vi "bumper.vi"() -> ()   [LabVIEW 2013]
uses:
  E:/All_Physics/PRISM/Abadines/bumper.ctl
  <vilib>/NXT/Block Support/NXT_InputPort.ctl
  <vilib>/NXT/Subs/MotorOutput.ctl
panel:
  out "F.  Right":bool
  out "F. Left":bool
  out "Output Ports (A & B) 8":T1=4 items=["Port A"=0, "Port B"=1, "Port C"=2, "Ports A & B"=4, "Ports A & C"=5, "Ports B & C"=6, "All Ports"=3]
  out "Output Port (All Ports) 2":T1=3 items=["Port A"=0, "Port B"=1, "Port C"=2, "Ports A & B"=4, "Ports A & C"=5, "Ports B & C"=6, "All Ports"=3]
  out "Output Ports (A & B) 7":T1=4 items=["Port A"=0, "Port B"=1, "Port C"=2, "Ports A & B"=4, "Ports A & C"=5, "Ports B & C"=6, "All Ports"=3]
  out "Output Ports (A & B) 6":T1=4 items=["Port A"=0, "Port B"=1, "Port C"=2, "Ports A & B"=4, "Ports A & C"=5, "Ports B & C"=6, "All Ports"=3]
  out "Output Ports (A & B) 5":T1=4 items=["Port A"=0, "Port B"=1, "Port C"=2, "Ports A & B"=4, "Ports A & C"=5, "Ports B & C"=6, "All Ports"=3]
  out "0 = Forward\n1 = F.  Left\n2 = F.  Right\n3 = B. Left\n4 = B. Right":i32
  in  "threshold steer":dbl=0.2
  out "norm dist":dbl
  out "right dist":i16
  out "left dist":i16
  out "Output Ports (A & B) 4":T1=4 items=["Port A"=0, "Port B"=1, "Port C"=2, "Ports A & B"=4, "Ports A & C"=5, "Ports B & C"=6, "All Ports"=3]
  out "Output Port (All Ports)":T1=3 items=["Port A"=0, "Port B"=1, "Port C"=2, "Ports A & B"=4, "Ports A & C"=5, "Ports B & C"=6, "All Ports"=3]
  out "Output Ports (A & B) 3":T1=4 items=["Port A"=0, "Port B"=1, "Port C"=2, "Ports A & B"=4, "Ports A & C"=5, "Ports B & C"=6, "All Ports"=3]
  out "Output Ports (A & B) 2":T1=4 items=["Port A"=0, "Port B"=1, "Port C"=2, "Ports A & B"=4, "Ports A & C"=5, "Ports B & C"=6, "All Ports"=3]
  out "Output Ports (A & B)":T1=4 items=["Port A"=0, "Port B"=1, "Port C"=2, "Ports A & B"=4, "Ports A & C"=5, "Ports B & C"=6, "All Ports"=3]
  out "Right Bumper":bool
  out "Left Bumper":bool
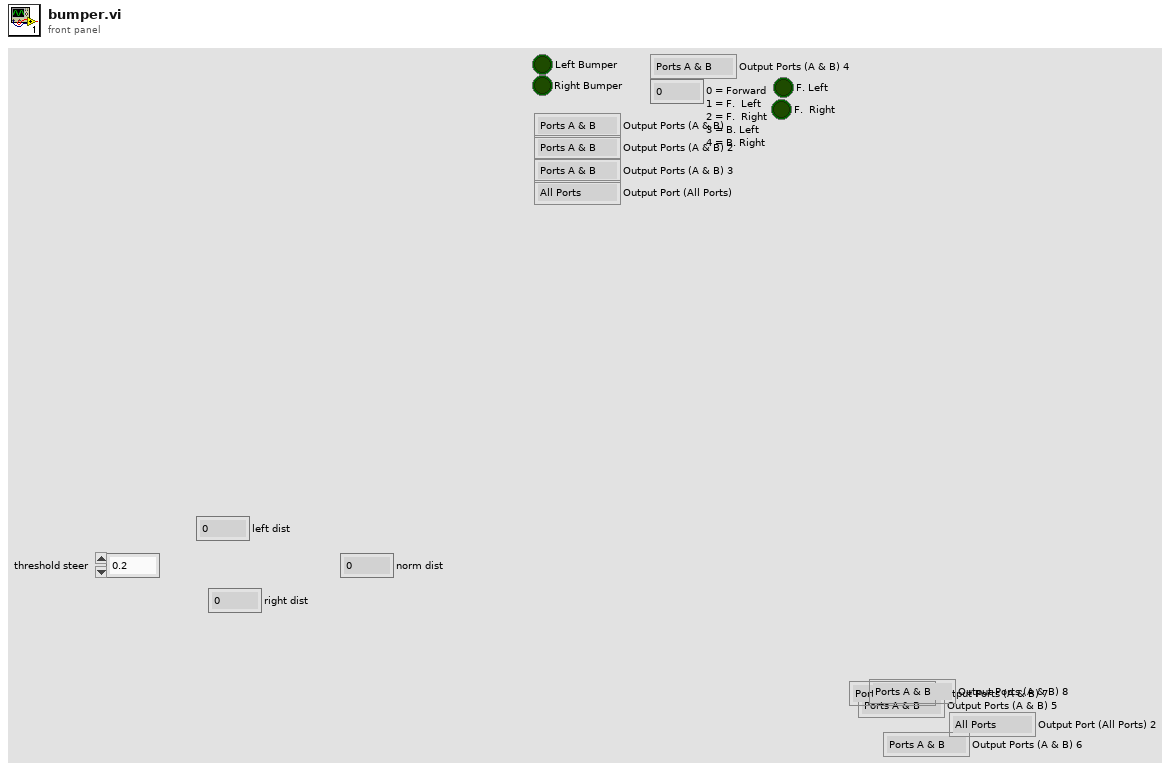
[diagram p1: front panel]
types:
  T1 = typedef "MotorOutput.ctl" = u8
  T2 = typedef "bumper.ctl" = enum16{"t", "b", "f"}
  T3 = typedef "NXT_InputPort.ctl" = u32
  T4 = typedef "LVHSConnector.ctl" = refnum<class "BrickReference.lvclass">
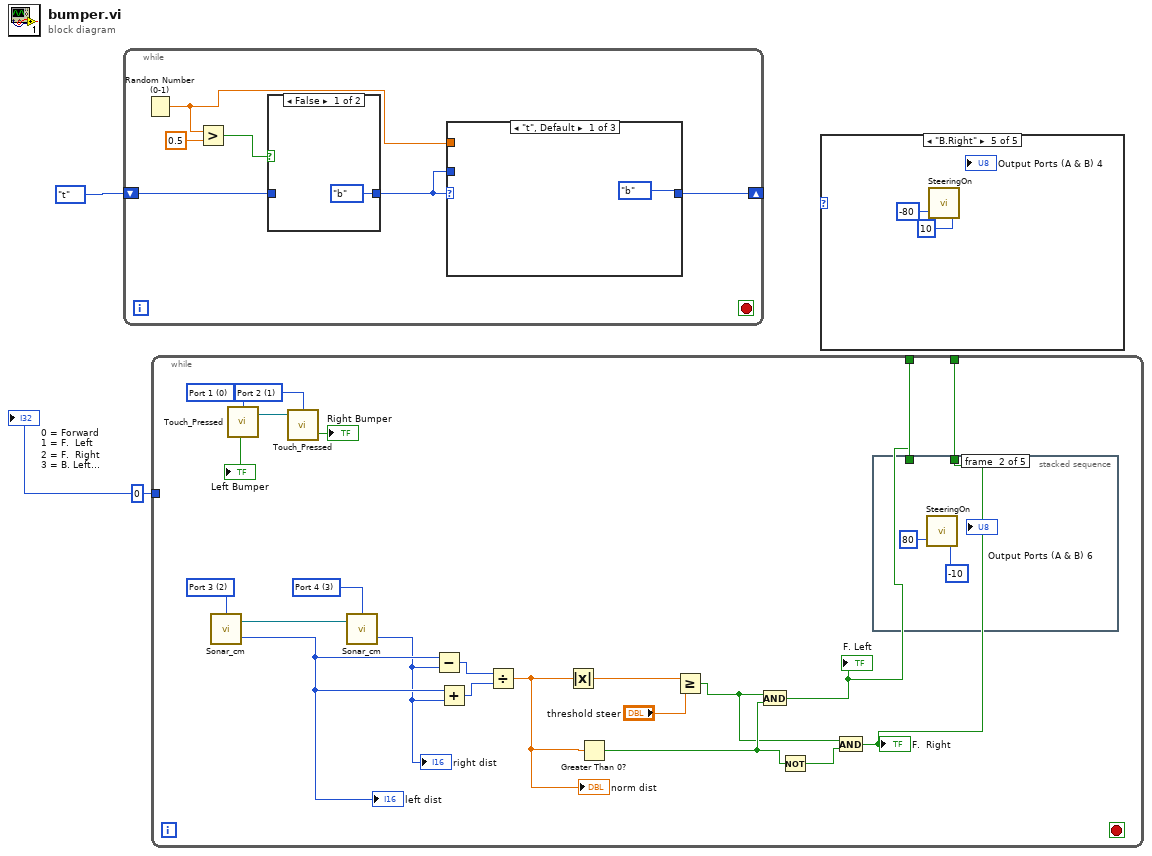
[diagram p0: block diagram]
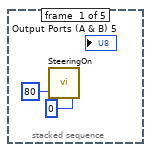
[diagram p2: hidden frame]
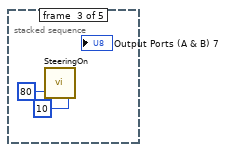
[diagram p3: hidden frame]
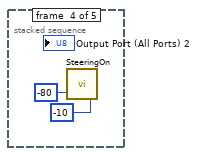
[diagram p4: hidden frame]
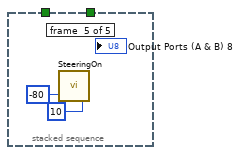
[diagram p5: hidden frame]
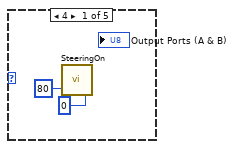
[diagram p6: hidden frame]
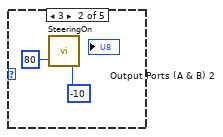
[diagram p7: hidden frame]
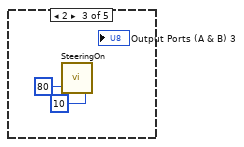
[diagram p8: hidden frame]
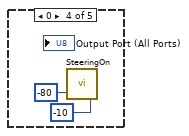
[diagram p9: hidden frame]
diagram:
  w3 = 0
  n1 = while {
    shift-right: [w10] -> _
    shift-left: bumper."t" -> [w7]
    stop <- _ stop-if-true
    n2 = Random Number (0-1)() -> (number: 0 to 1=w5:dbl)
    n3 = Greater?(x=w5, y=0.5) -> (0:w8:bool)
    n4 = case shown="False" w8 {
      tunnel: w7 -> [_ w12]
      tunnel: [bumper."b" w12] -> w6
      frame False {
      }
      frame True {
      }
    }
    n5 = case shown="\"t\", Default" w6 {
      tunnel: w6 -> [_ w14 _]
      tunnel: [bumper."b" w14 _] -> w10
      tunnel: w5 -> [_ _ _]
      frame "t", Default {
      }
      frame "b" {
      }
      frame "f" {
      }
    }
  }
  n6 = while {
    tunnel: w3 -> [_]
    tunnel: [w19] -> w2
    tunnel: [w15] -> w1
    stop <- _ stop-if-true
    w28 = T3 3 items=["Port 1", "Port 2", "Port 3", "Port 4"] ("Port (Port 4)")
    w29 = T3 2 items=["Port 1", "Port 2", "Port 3", "Port 4"] ("Port (Port 4)")
    w33 = T3 1 items=["Port 1", "Port 2", "Port 3", "Port 4"] ("Port (Port 1)")
    w34 = T3 0 items=["Port 1", "Port 2", "Port 3", "Port 4"] ("Port (Port 1)")
    n7 = call <vilib>:"Sonar_cm.vi"("Port (Port 4)"=w29) -> ("Distance (cm)"=w26:i16, "NXT/EV3"=w27:T4)  [unwired: 2 in]
    "left dist" <- w26
    n8 = call <vilib>:"Touch_Pressed.vi"("Port (Port 1)"=w34) -> ("Yes / No"=→"Left Bumper":bool, "NXT/EV3"=w30:T4)  [unwired: 2 in]
    n9 = call <vilib>:"Touch_Pressed.vi"("NXT/EV3"=w30, "Port (Port 1)"=w33) -> ("Yes / No"=→"Right Bumper":bool)  [unwired: 1 in, 1 out]
    n10 = call <vilib>:"Sonar_cm.vi"("NXT/EV3"=w27, "Port (Port 4)"=w28) -> ("Distance (cm)"=w25:i16)  [unwired: 1 in, 1 out]
    "right dist" <- w25
    n11 = Subtract(x=w26, y=w25) -> (x-y=w24:i16)
    n12 = Add(x=w26, y=w25) -> (x+y=w23:i16)
    n13 = Divide(x=w24, y=w23) -> (x/y=w20:dbl)
    "norm dist" <- w20
    n14 = Absolute Value(x=w20) -> (abs(x)=w22:dbl)
    n15 = Greater Than 0?(x=w20) -> (x > 0?=w18:bool)
    n16 = Greater Or Equal?(x=w22, y="threshold steer") -> (x >= y?=w17:bool)
    n17 = And(x=w17, y=w18) -> (x .and. y?=w19:bool)
    "F. Left" <- w19
    n18 = Not(x=w18) -> (.not. x?=w16:bool)
    n19 = And(x=w17, y=w16) -> (x .and. y?=w15:bool)
    "F.  Right" <- w15
  }
  n20 = case shown="\"B.Right\"" {
    selector: _ -> [_ _ _ _ _]
    frame 4 {
      n21 = call <vilib>:"SteeringOn.vi"("Power (75)"=80, "Steering (100)"=0) -> ()  [unwired: 2 in, 1 out]
    }
    frame 3 {
      n22 = call <vilib>:"SteeringOn.vi"("Power (75)"=80, "Steering (100)"=-10) -> ()  [unwired: 2 in, 1 out]
    }
    frame 2 {
      n23 = call <vilib>:"SteeringOn.vi"("Power (75)"=80, "Steering (100)"=10) -> ()  [unwired: 2 in, 1 out]
    }
    frame 0 {
      n24 = call <vilib>:"SteeringOn.vi"("Power (75)"=-80, "Steering (100)"=-10) -> ()  [unwired: 2 in, 1 out]
    }
    frame 1 {
      n25 = call <vilib>:"SteeringOn.vi"("Power (75)"=-80, "Steering (100)"=10) -> ()  [unwired: 2 in, 1 out]
    }
  }
  n26 = stacked-sequence {
    tunnel: w2 -> [_ _ _ _ _]
    tunnel: w1 -> [_ _ _ _ _]
    frame #0 {
      n27 = call <vilib>:"SteeringOn.vi"("Power (75)"=80, "Steering (100)"=0) -> ()  [unwired: 2 in, 1 out]
    }
    frame #1 {
      n28 = call <vilib>:"SteeringOn.vi"("Power (75)"=80, "Steering (100)"=-10) -> ()  [unwired: 2 in, 1 out]
    }
    frame #2 {
      n29 = call <vilib>:"SteeringOn.vi"("Power (75)"=80, "Steering (100)"=10) -> ()  [unwired: 2 in, 1 out]
    }
    frame #3 {
      n30 = call <vilib>:"SteeringOn.vi"("Power (75)"=-80, "Steering (100)"=-10) -> ()  [unwired: 2 in, 1 out]
    }
    frame #4 {
      n31 = call <vilib>:"SteeringOn.vi"("Power (75)"=-80, "Steering (100)"=10) -> ()  [unwired: 2 in, 1 out]
    }
  }
  "0 = Forward\n1 = F.  Left\n2 = F.  Right\n3 = B. Left\n4 = B. Right" <- w3
